vi "Initialize Section Page.vi"(7 "Properties":refnum<k24>, 8 "error in":errorcluster, 11 "Node Ptr":T1 format="%.0x") -> (0 "error out":errorcluster, 3 "Node Ptr out":T1=18446744073709551615 format="%.0x")   [LabVIEW 2026]
uses:
  C:/Program Files/National Instruments/VeriStand 2026/NationalInstruments.VeriStand.Controls.dll
  Program Files/National Instruments/VeriStand 2026/NationalInstruments.VeriStand.Controls.dll
  C:/Program Files/National Instruments/LabVIEW 2025/ProjectTemplates/Source/NI Veristand/Custom Device/Template Files/NationalInstruments.VeriStand.DummyPlugin.dll
  Program Files/National Instruments/LabVIEW 2025/ProjectTemplates/Source/NI Veristand/Custom Device/Template Files/NationalInstruments.VeriStand.DummyPlugin.dll
  <vilib>/NI VeriStand/Custom Device API/Custom Device Item Ref.ctl
  <vilib>/NI VeriStand/Custom Device API/Custom Device API.lvlib
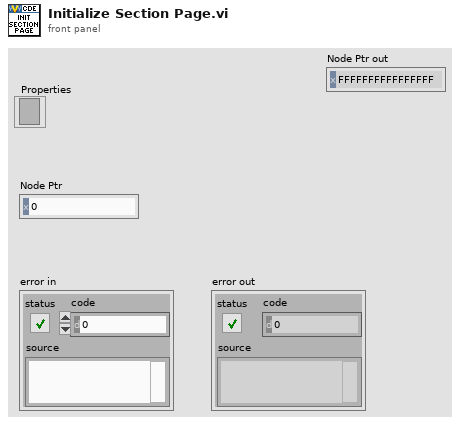
[diagram p1: front panel]
types:
  T1 = typedef "Custom Device API.lvlib/Custom Device Item Ref.ctl" = u64
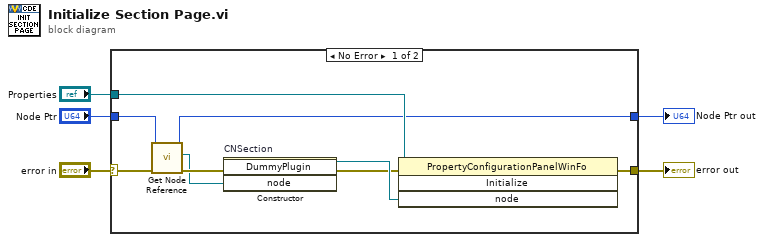
[diagram p0: block diagram]
diagram:
  n1 = case shown="No Error" "error in" {
    selector: "error in" -> [w7 w15]
    tunnel: "Properties" -> [w14 _]
    tunnel: [w12 w15] -> w4
    tunnel: "Node Ptr" -> [w8 w16]
    tunnel: [w6 w16] -> w1
    frame No Error {
      n2 = call "Get Node Reference.vi"("error in"=w7, "Node Ptr"=w8) -> ("error out"=w10:errorcluster, "BaseNodeType"=w9:refnum<k24>, "Node Ptr"=w6:T1)  [unwired: 6 in, 1 out]
      n3 = constructor on="CNSection" class="DummyPlugin"(error in=w10, "node"=w9) -> (reference out=w13:refnum<k24>, error out=w11:errorcluster)  [unwired: 2 in, 2 out]
      n4 = invoke class="PropertyConfigurationPanelWinFo" method="Initialize"(reference=w14, error in=w11, "node"=w13) -> (error out=w12:errorcluster)  [unwired: 1 in, 3 out]
    }
    frame Error {
    }
  }
  "error out" <- w4
  "Node Ptr out" <- w1
